vi "Configure Pressure Control.vi"(8 "error in":errorcluster, 11 "Red-y Read Write CFG in":refnum<class "Red-y Pressure Control CFG.lvclass">) -> (0 "error out":errorcluster, 3 "Red-y Read Write CFG out":refnum<class "Red-y Pressure Control CFG.lvclass">)   [LabVIEW 2023, in "Red-y Pressure Control CFG.lvclass"]
uses:
  Red-y Pressure Control CFG.lvclass
  Configuration/Configuration JSON/Configuration JSON Base/CFG JSON.lvclass/CFG JSON.ctl
  <userlib>/_OpenG.lib/lvdata/lvdata.llb/Type Descriptor Enumeration__ogtk.ctl
  65c23efe-83e5-47bf-b2b0-76bae52f3ad0.vi
  <vilib>/JDP Science/JSONtext/JSON text to Variant.vi
  <vilib>/JDP Science/JSONtext/LVClass Serializer/JSONtext LVClass Serializer.lvclass
  Red-y Pressure Control CFG.lvclass/Red-y Pressure Control CFG.ctl
  Configuration/Configuration JSON/Configuration JSON Base/CFG JSON.lvclass
  <userlib>/_OpenG.lib/lvdata/lvdata.llb/openg_variant.lvlib
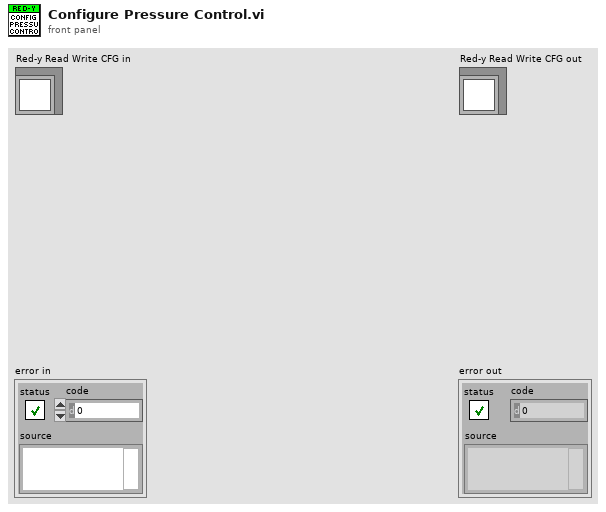
[diagram p1: front panel]
types:
  T1 = typedef "openg_variant.lvlib/Type Descriptor Enumeration__ogtk.ctl" = enum8{"<Null>", "I8", "I16", "I32", "I64", "U8", "U16", "U32", "U64", "SGL", "DBL", "EXT", "CSG", "CDB", "CXT", "0x0F", "0x10", "0x11", "0x12", "0x13", "0x14", "Enum U8", "Enum U16", "Enum U32", "Enum U64", "SGL PQ", "DBL PQ", "EXT PQ", "CSG PQ", "CDB PQ", "CXT PQ", "0x1F", "0x20", "Boolean", "0x22", "0x23", "0x24", "0x25", "0x26", "0x27", "0x28", "0x29", "0x2A", "0x2B", "0x2C", "0x2D", "0x2E", "0x2F", "String", "0x31", "Path", "Pict", "0x34", "0x35", "0x36", "DAQ", "0x38", "0x39", "0x3A", "0x3B", "0x3C", "0x3D", "0x3E", "0x3F", "Array", "0x41", "0x42", "0x43", "0x44", "0x45", "0x46", "0x47", "0x48", "0x49", "0x4A", "0x4B", "0x4C", "0x4D", "0x4E", "0x4F", "Cluster", "0x51", "0x52", "Variant", "Waveform", "0x55", "0x56", "0x57", "0x58", "0x59", "0x5A", "0x5B", "0x5C", "0x5D", "0x5E", "Fixed Point", "0x60", "0x61", "0x62", "0x63", "0x64", "0x65", "0x66", "0x67", "0x68", "0x69", "0x6A", "0x6B", "0x6C", "0x6D", "0x6E", "0x6F", "Refnum", "0x71", "0x72", "Set Collection", "Map Collection"}
  T2 = enum16{"0..20 mA / 0..5 V", "4..20 mA / 1..5 V", "4..20 mA / 1..5 V2", "0..20 mA / 0..10 V", "0..20 mA / 2..10 V", "User Defined"}
  T3 = enum16{"Automatic", "Digital Setpoint", "Analog Setpoint"}
  T4 = cluster{"Control Mode":string, "Pressure Unit":string, "Signal Type AI":string, "Scaling Pressure Min":sgl, "Scaling Pressure Max":sgl, "Flow Limiting":sgl, "Pressure Control Mode":string, "Flow Limiting Active":bool, "Pressure Setpoint":sgl}
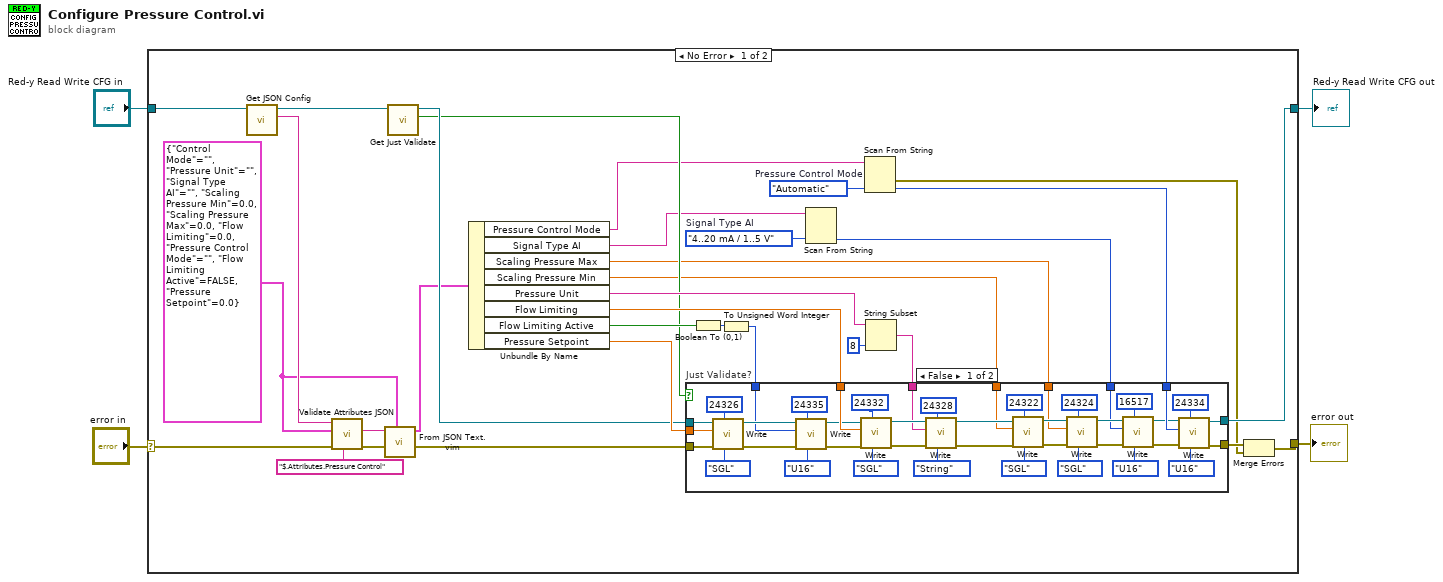
[diagram p0: block diagram]
diagram:
  n1 = case shown="No Error" "error in" {
    selector: "error in" -> [w10 w82]
    tunnel: [w20 w82] -> w3
    tunnel: [w31 w81] -> w1
    tunnel: "Red-y Read Write CFG in" -> [w36 w81]
    frame No Error {
      w13 = T2."4..20 mA / 1..5 V"  # Signal Type AI
      w25 = T3."Automatic"  # Pressure Control Mode
      w6 = T4 {"Control Mode"="", "Pressure Unit"="", "Signal Type AI"="", "Scaling Pressure Min"=0.0, "Scaling Pressure Max"=0.0, "Flow Limiting"=0.0, "Pressure Control Mode"="", "Flow Limiting Active"=FALSE, "Pressure Setpoint"=0.0}
      n2 = call "Get JSON Config.vi"("CFG Base in"=w36) -> ("<JSON>Config>"=w9:string, "CFG Base out"=w35:refnum<class "Red-y Pressure Control CFG.lvclass">)  [unwired: 9 in]
      n3 = call "Validate Attributes JSON.vi"("$Path"="$.Attributes.Pressure Control", "error in"=w10, "Cluster in"=w6, "<JSON>"=w9) -> ("error out"=w11:errorcluster, "<JSON>"=w8:string)  [unwired: 6 in]
      n4 = call "From JSON Text.vim"("Data Type and Default Value"=w6, "error in (no error)"=w11, "JSON"=w8) -> ("error out"=w30:errorcluster, "Data out"=w7:T4)  [unwired: 7 in]
      n5 = call "Get Just Validate.vi"("CFG JSON Base in"=w35) -> ("Just Validate"=w21:bool, "CFG JSON Base out"=w22:refnum<class "Red-y Pressure Control CFG.lvclass">)  [unwired: 9 in]
      n6 = Unbundle By Name(w7) -> ("Pressure Control Mode"=w18:string, "Signal Type AI"=w14:string, "Scaling Pressure Max"=w15:sgl, "Scaling Pressure Min"=w16:sgl, "Pressure Unit"=w33:string, "Flow Limiting"=w24:sgl, "Flow Limiting Active"=w27:bool, "Pressure Setpoint"=w29:sgl)
      n7 = Boolean To (0,1)(Boolean=w27) -> (0, 1=w28:i16)
      n8 = To Unsigned Word Integer(number=w28) -> (unsigned 16bit integer=w26:u16)
      n9 = Scan From String(input string=w14, default 1=w13) -> (output 1=w12:T2)  [unwired: 3 in, 3 out]
      n10 = Scan From String(input string=w18, default 1=w25) -> (error out=w19:errorcluster, output 1=w17:T3)  [unwired: 3 in, 2 out]
      n11 = String Subset(string=w33, length (rest)=8 ("length (rest)")) -> (substring=w23:string)  [unwired: 1 in]
      n12 = case "Just Validate?" shown="False" w21 {
        tunnel: w22 -> [w78 w80]
        tunnel: w30 -> [w77 w79]
        tunnel: [w58 w79] -> w32
        tunnel: [w57 w80] -> w31
        tunnel: w29 -> [w70 _]
        tunnel: w26 -> [w69 _]
        tunnel: w24 -> [w64 _]
        tunnel: w23 -> [w61 _]
        tunnel: w17 -> [w56 _]
        tunnel: w16 -> [w51 _]
        tunnel: w15 -> [w48 _]
        tunnel: w12 -> [w37 _]
        frame False {
          n13 = call "Write.vi"("Type"=Type_Descriptor_Enumeration__ogtk."SGL", "Register"=u16 24326, "error in"=w77, "Data"=w70, "Red-y Pressure Control CFG in"=w78) -> ("error out"=w74:errorcluster, "Red-y Pressure Control CFG out"=w73:refnum<class "Red-y Pressure Control CFG.lvclass">)  [unwired: 5 in]
          n14 = call "Write.vi"("Type"=Type_Descriptor_Enumeration__ogtk."U16", "Register"=u16 24335, "error in"=w74, "Data"=w69, "Red-y Pressure Control CFG in"=w73) -> ("error out"=w55:errorcluster, "Red-y Pressure Control CFG out"=w54:refnum<class "Red-y Pressure Control CFG.lvclass">)  [unwired: 5 in]
          n15 = call "Write.vi"("Type"=Type_Descriptor_Enumeration__ogtk."SGL", "Register"=u16 24332, "error in"=w55, "Data"=w64, "Red-y Pressure Control CFG in"=w54) -> ("error out"=w75:errorcluster, "Red-y Pressure Control CFG out"=w76:refnum<class "Red-y Pressure Control CFG.lvclass">)  [unwired: 5 in]
          n16 = call "Write.vi"("Type"=Type_Descriptor_Enumeration__ogtk."String", "Register"=u16 24328, "error in"=w75, "Data"=w61, "Red-y Pressure Control CFG in"=w76) -> ("error out"=w53:errorcluster, "Red-y Pressure Control CFG out"=w52:refnum<class "Red-y Pressure Control CFG.lvclass">)  [unwired: 5 in]
          n17 = call "Write.vi"("Type"=Type_Descriptor_Enumeration__ogtk."SGL", "Register"=u16 24322, "error in"=w53, "Data"=w51, "Red-y Pressure Control CFG in"=w52) -> ("error out"=w50:errorcluster, "Red-y Pressure Control CFG out"=w49:refnum<class "Red-y Pressure Control CFG.lvclass">)  [unwired: 5 in]
          n18 = call "Write.vi"("Type"=Type_Descriptor_Enumeration__ogtk."SGL", "Register"=u16 24324, "error in"=w50, "Data"=w48, "Red-y Pressure Control CFG in"=w49) -> ("error out"=w43:errorcluster, "Red-y Pressure Control CFG out"=w41:refnum<class "Red-y Pressure Control CFG.lvclass">)  [unwired: 5 in]
          n19 = call "Write.vi"("Type"=Type_Descriptor_Enumeration__ogtk."U16", "Register"=u16 16517, "error in"=w43, "Data"=w37, "Red-y Pressure Control CFG in"=w41) -> ("error out"=w42:errorcluster, "Red-y Pressure Control CFG out"=w40:refnum<class "Red-y Pressure Control CFG.lvclass">)  [unwired: 5 in]
          n20 = call "Write.vi"("Type"=Type_Descriptor_Enumeration__ogtk."U16", "Register"=u16 24334, "error in"=w42, "Data"=w56, "Red-y Pressure Control CFG in"=w40) -> ("error out"=w58:errorcluster, "Red-y Pressure Control CFG out"=w57:refnum<class "Red-y Pressure Control CFG.lvclass">)  [unwired: 5 in]
        }
        frame True {
        }
      }
      n21 = Merge Errors(w32, w19) -> (w20:errorcluster)
    }
    frame Error {
    }
  }
  "error out" <- w3
  "Red-y Read Write CFG out" <- w1
